vi "Phasor Compute f(tau) & Zeros.vi"(0 "f(tau) Graph Refnum":refnum<vi>, 1 "Phasor Graph Refnum":refnum<vi>, 5 "Phasor Parameters":T1={"Display Parameters"={"# Points"=0, "Ramp Type"=enum."Linear", "Type of Series"=enum."1-Exp Decays", "Min tau"=0.0, "Max tau"=0.0, "Include 0"=FALSE, "Include Infinity"=FALSE}, "Phasor Parameters"={"Harmonic Frequency"=0.0, "Use f* = 1/D Frequency"=FALSE, "Calibrated Phasor"=FALSE, "Calibration Lifetime"=1e-09, "Phasor Calculation"=enum."Direct Sum", "SEPL Type"=enum."UC", "# Gates"=1.0, "Square Gate Width"=1e-09, "Show Ticks"=FALSE}, "Decay & IRF Parameters"={"Lifetime"=0.0, "IRF Offset"=0.0, "IRF Period"=0.0, "Normalized Decays"=FALSE, "IRF Model"=enum."Dirac", "IRF Parameter 1"=0.0}, "Gate Parameters"={"First Gate Start"=0.0, "Use Gate Center"=FALSE, "Gate Width"=0.0, "Gate Step"=0.0, "# Gates"=0.0, "Gate Type"=enum."Square", "Edge Width"=0.0, "Top Slope"=0.0, "Reversed Sawtooth?"=FALSE, "Analytical Computation"=FALSE, "Integration"=enum."Item 0", "Tolerance"=1.0, "# Steps"=1.0, "Type of User-defined Function"=enum."Gate", "Use Gate Step"=FALSE}, "Detector Parameters"={"Frames/Image"=0, "Gates/Frame"=0, "Bits/Frame"=0, "Multiplicity"=0, "Incident Signal"=0.0, "Poisson Signal"=FALSE}} {"Detector Parameters"."Frames/Image" min=1; "Detector Parameters"."Multiplicity" min=0; "Detector Parameters"."Bits/Frame" min=1; "Detector Parameters"."Gates/Frame" min=1; "Gate Parameters"."# Steps" min=0.0; "Gate Parameters"."Tolerance" min=0.0; "Gate Parameters"."Top Slope" min=0.0; "Gate Parameters"."Edge Width" min=0.0; "Gate Parameters"."Gate Step" min=0.0; "Gate Parameters"."# Gates" min=0.0 step=1.0; "Gate Parameters"."Gate Width" min=0.0; "Decay & IRF Parameters"."Lifetime" min=0.0; "Decay & IRF Parameters"."IRF Period" min=0.0; "Phasor Parameters"."Square Gate Width" min=0.0; "Phasor Parameters"."# Gates" min=0.0; "Phasor Parameters"."Calibration Lifetime" min=0.0; "Phasor Parameters"."Harmonic Frequency" min=0.0; "Display Parameters"."Min tau" min=0.0; "Display Parameters"."Max tau" min=0.0; "Display Parameters"."# Points" min=1 step=1}, 7 "Linear Coefficients":cluster{"u":dbl, "v":dbl}, 11 "Error In":errorcluster, 12 "Use Cursor":bool) -> (4 "Numerical Solution 1":dbl[unit], 6 "Numerical Solution 2":dbl[unit], 8 "Analytical Solution 1":dbl[unit], 10 "Analytical Solution 2":dbl[unit], 15 "Error Out":errorcluster)   [LabVIEW 2021, in "Phasor.lvlib"]
uses:
  Phasor.lvlib
  Phasor SEPL Parameters.ctl
  Phasor Explorer Display Parameters.ctl
  Phasor Type of Series.ctl
  Phasor Explorer Phasor Parameters.ctl
  Phasor Calculation Type.ctl
  Phasor SEPL Type.ctl
  Phasor Explorer Decay Parameters.ctl
  Phasor IRF Model.ctl
  Phasor Explorer Gate Parameters.ctl
  Phasor Gate Type.ctl
  Phasor Type of User-defined Function.ctl
  Phasor Explorer Detector Parameters.ctl
  Phasor Explorer f(tau) [SEPL Intersections].vi
  <vilib>/gmath/zero.llb/Find All Zeros of f(x) (VI).vi
  <vilib>/ErrorRing/Error Ring.xnode
  Image/Image.lvlib
  <vilib>/gmath/NI_Gmath.lvlib
  Phasor Explorer.lvlib
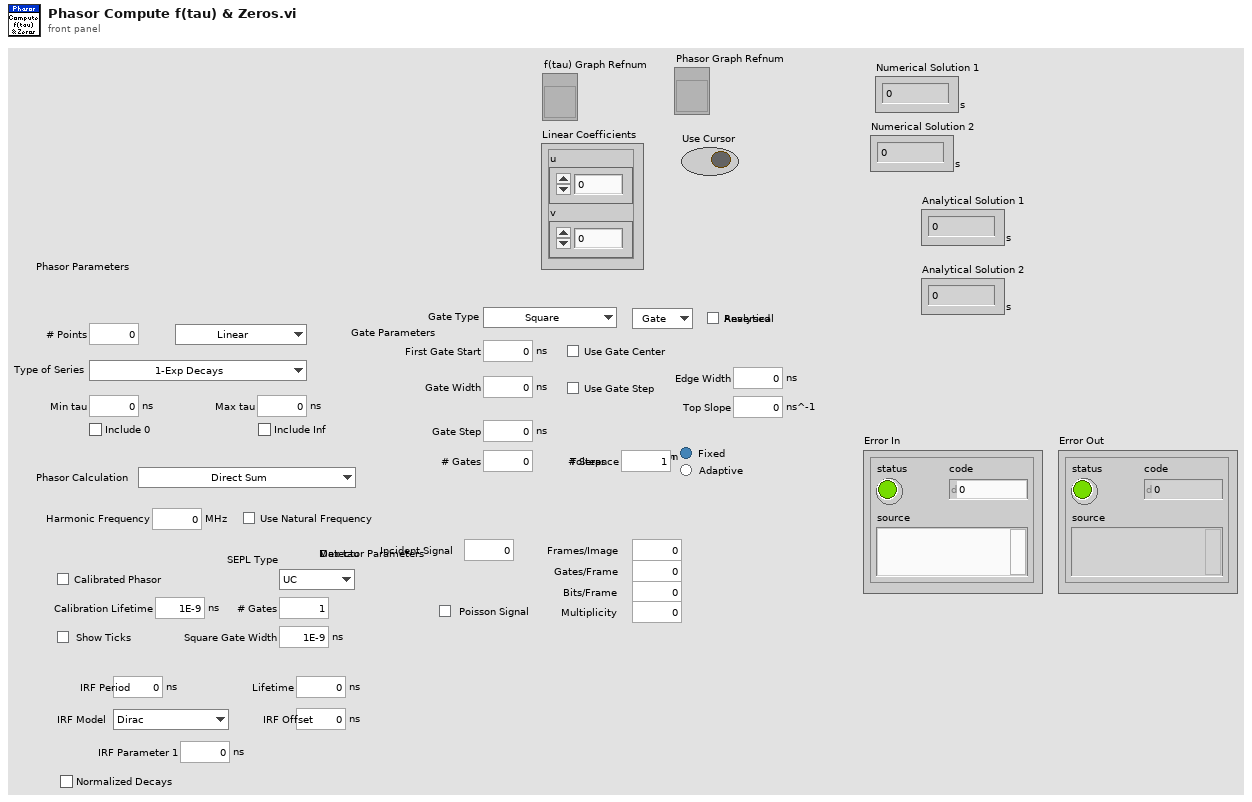
[diagram p1: front panel]
types:
  T1 = typedef "Phasor.lvlib/Phasor SEPL Parameters.ctl" = cluster{"Display Parameters":T2, "Phasor Parameters":T4, "Decay & IRF Parameters":T7, "Gate Parameters":T9, "Detector Parameters":T12}
  T2 = typedef "Phasor Explorer.lvlib/Phasor Explorer Display Parameters.ctl" = cluster{"# Points":i32, "Ramp Type":enum16{"Linear", "Logarithmic"}, "Type of Series":T3, "Min tau":dbl[unit], "Max tau":dbl[unit], "Include 0":bool, "Include Infinity":bool}
  T3 = typedef "Phasor.lvlib/Phasor Type of Series.ctl" = enum16{"1-Exp Decays", "Linear Combination of 1-Exp"}
  T4 = typedef "Phasor Explorer.lvlib/Phasor Explorer Phasor Parameters.ctl" = cluster{"Harmonic Frequency":dbl[unit], "Use f* = 1/D Frequency":bool, "Calibrated Phasor":bool, "Calibration Lifetime":dbl[unit], "Phasor Calculation":T5, "SEPL Type":T6, "# Gates":dbl, "Square Gate Width":dbl[unit], "Show Ticks":bool}
  T5 = typedef "Phasor.lvlib/Phasor Calculation Type.ctl" = enum16{"Direct Sum", "Analytical Formula"}
  T6 = typedef "Phasor.lvlib/Phasor SEPL Type.ctl" = enum16{"UC", "L_N", "L_N[W]", "L_X"}
  T7 = typedef "Phasor Explorer.lvlib/Phasor Explorer Decay Parameters.ctl" = cluster{"Lifetime":dbl[unit], "IRF Offset":dbl[unit], "IRF Period":dbl[unit], "Normalized Decays":bool, "IRF Model":T8, "IRF Parameter 1":dbl[unit]}
  T8 = typedef "Phasor.lvlib/Phasor IRF Model.ctl" = enum16{"Dirac", "Exponential"}
  T9 = typedef "Phasor Explorer.lvlib/Phasor Explorer Gate Parameters.ctl" = cluster{"First Gate Start":dbl[unit], "Use Gate Center":bool, "Gate Width":dbl[unit], "Gate Step":dbl[unit], "# Gates":dbl, "Gate Type":T10, "Edge Width":dbl[unit], "Top Slope":dbl[unit], "Reversed Sawtooth?":bool, "Analytical Computation":bool, "Integration":enum32{"Item 0", "Item 1"}, "Tolerance":dbl, "# Steps":dbl, "Type of User-defined Function":T11, "Use Gate Step":bool}
  T10 = typedef "Phasor.lvlib/Phasor Gate Type.ctl" = enum16{"Square", "Finite Edge Square", "Finite Edge, Tilted Top Square", "Triangle", "Sawtooth", "User-defined"}
  T11 = typedef "Phasor.lvlib/Phasor Type of User-defined Function.ctl" = enum16{"Gate", "IRF"}
  T12 = typedef "Phasor Explorer.lvlib/Phasor Explorer Detector Parameters.ctl" = cluster{"Frames/Image":i32, "Gates/Frame":i32, "Bits/Frame":i32, "Multiplicity":i32, "Incident Signal":dbl, "Poisson Signal":bool}
  T13 = typedef "LVCursorListTypeDef.ctl" = cluster{"Name":string, "Color":u32, "Style":u8, "Point Style":u8, "Name Visible":bool, "Allow Drag":bool, "Cursor Mode":u32, "Plot":i32, "Index":i32, "Position":cluster{"X":dbl, "Y":dbl}, "X Scale":u32, "Y Scale":u32, "Watch Plots":i32[], "Watch All Plots":bool, "Plot Area":i32, "Label Offset":cluster{"X":dbl, "Y":dbl}}[]
  T14 = cluster{"Name":string, "Color":u32, "Style":u8, "Point Style":u8, "Name Visible":bool, "Allow Drag":bool, "Cursor Mode":u32, "Plot":i32, "Index":i32, "Position":cluster{"X":dbl, "Y":dbl}, "X Scale":u32, "Y Scale":u32, "Watch Plots":i32[], "Watch All Plots":bool, "Plot Area":i32, "Label Offset":cluster{"X":dbl, "Y":dbl}}
  T15 = typedef "Phasor.lvlib/Phasor Data for SEPL Intersections.ctl" = cluster{"Linear Coefficients":cluster{"u":dbl, "v":dbl}, "Decay Definition":T16, "Gates Definitions":T17, "iw":cdb, "Phasor Calculation":T5}
  T16 = typedef "Phasor.lvlib/Phasor Decay Definiton.ctl" = cluster{"offset: t0":ext, "period: T":ext, "lifetime: tau":ext, "Incident Signal: I":ext, "Normalized Decays":bool, "IRF Model":T8, "IRF Parameter 1":ext, "Poisson Signal":bool}
  T17 = typedef "Phasor.lvlib/Phasor Gate Definitions.ctl" = cluster{"First Gate: t1":ext, "Gate Width: W":ext, "Gate Step: d":ext, "# Gates: G":ext, "Use Gate Center":bool, "Frames/Image: F":i32, "Gates/Frame: L":i32, "Bits/Frame: q":i32, "Multiplicity: p":i32, "Gate Type":T10, "Gate Edge s":ext, "Gate Top Slope":ext, "Reversed Sawtooth?":bool, "Computation":bool, "User-defined Gate":T18, "Tolerance":ext, "Integration":enum32{"Item 0", "Item 1"}, "# Steps":ext, "Type of User-defined Function":enum32{"Gate", "IRF"}}
  T18 = typedef "XY Graph Add-Ons.lvlib/XY Plot Data.ctl" = cluster{"X Array":dbl[], "Y Array":dbl[]}
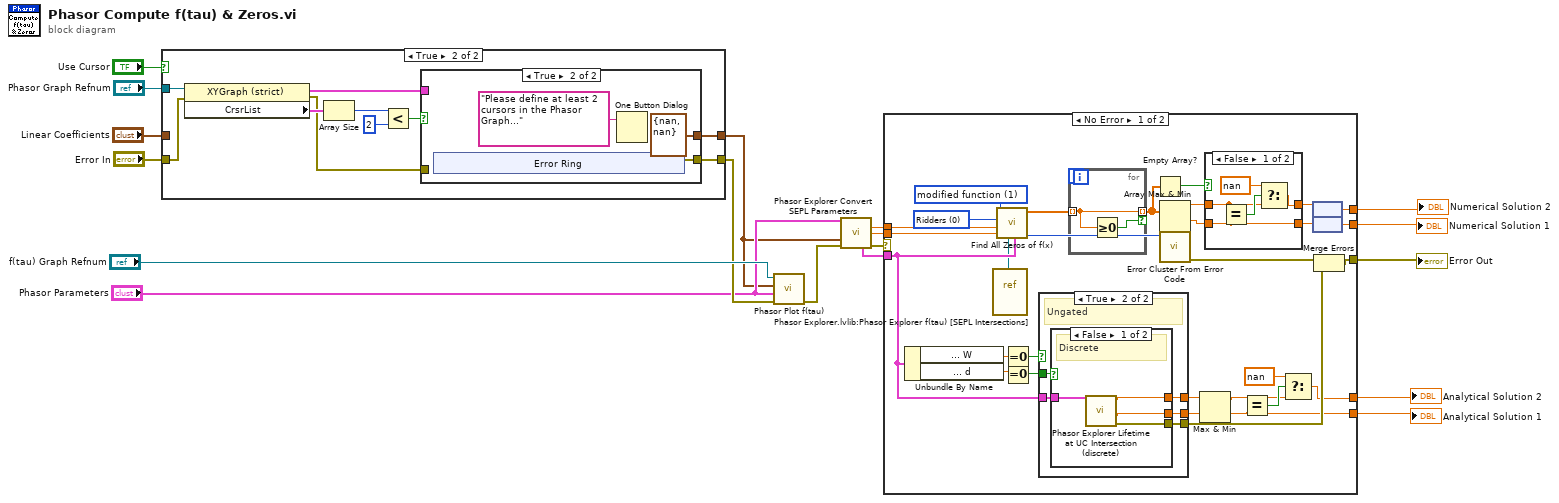
[diagram p0: block diagram]
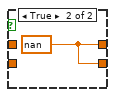
[diagram p2: hidden frame]
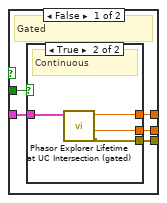
[diagram p3: hidden frame]
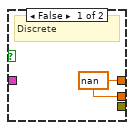
[diagram p4: hidden frame]
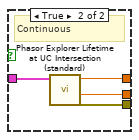
[diagram p5: hidden frame]
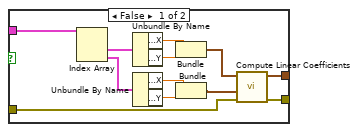
[diagram p8: hidden frame]
diagram:
  n1 = case shown="True" "Use Cursor" {
    tunnel: "Phasor Graph Refnum" -> [_ w29]
    tunnel: [w20 w24] -> w5
    tunnel: "Linear Coefficients" -> [w20 _]
    tunnel: "Error In" -> [w19 w23]
    tunnel: [w19 w21] -> w13
    frame False {
    }
    frame True {
      n2 = property class="XYGraph (strict)"(reference=w29, error in=w23) -> (error out=w22:errorcluster, "CrsrList"=w25:T13)  [unwired: 1 out]
      n3 = Array Size(array=w25) -> (size(s)=w28:i32)
      n4 = Less?(x=w28, y=2) -> (x < y?=w26:bool)
      n5 = case shown="True" w26 {
        tunnel: w25 -> [w41 _]
        tunnel: [w33 cluster{"u":dbl, "v":dbl} {"u"=nan, "v"=nan} ("Linear Coefficients")] -> w24
        tunnel: w22 -> [w31 _]
        tunnel: [w30 w42] -> w21
        frame False {
          n6 = Index Array(array=w41) -> (element #1=w40:T14, element #2=w39:T14)  [unwired: 2 in]
          n7 = Unbundle By Name(w40) -> ("Position.X"=w38:dbl, "Position.Y"=w37:dbl)
          n8 = Unbundle By Name(w39) -> ("Position.X"=w35:dbl, "Position.Y"=w34:dbl)
          n9 = Bundle("X"=w38, "Y"=w37) -> (w36:cluster{"X":dbl, "Y":dbl})  [unwired: 1 in]
          n10 = Bundle("X"=w35, "Y"=w34) -> (w32:cluster{"X":dbl, "Y":dbl})  [unwired: 1 in]
          n11 = call "Compute Linear Coefficients.vi"("Error In"=w31, "Point 2"=w32, "Point 1"=w36) -> ("Error Out"=w30:errorcluster, "Linear Coefficients"=w33:cluster{"u":dbl, "v":dbl})  [unwired: 7 in]
        }
        frame True {
          n12 = xnode "Error Ring"() -> ("error out"=w42:errorcluster)
          n13 = One Button Dialog(message="Please define at least 2 cursors in the Phasor Graph...") -> ()  [unwired: 1 in, 1 out]
        }
      }
    }
  }
  n14 = call "Phasor Plot f(tau).vi"("error in (no error)"=w13, "Phasor Parameters"="Phasor Parameters", "Linear Coefficients"=w5, "XYGraph in"="f(tau) Graph Refnum") -> ("error out"=w11:errorcluster)  [unwired: 7 in]
  n15 = call "Phasor Explorer Convert SEPL Parameters.vi"("Phasor Parameters"="Phasor Parameters", "Linear Coefficients"=w5, "Error In"=w11) -> ("Min tau"=w9:dbl, "Max tau"=w8:dbl, "Data for Pseudo UC Intersections"=w7:T15, "Error Out"=w10:errorcluster)  [unwired: 7 in, 2 out]
  n16 = case shown="No Error" w10 {
    selector: w10 -> [_ w110]
    tunnel: w9 -> [w76 _]
    tunnel: w8 -> [w75 _]
    tunnel: w7 -> [w66 _]
    tunnel: [w65 w110] -> w6
    tunnel: [w72 _] -> w4
    tunnel: [w71 _] -> w3
    tunnel: [w53 _] -> w2
    tunnel: [w49 _] -> w1
    frame No Error {
      w77 = u16 1 items=["fixed function", "modified function"] ("step type")
      w78 = u16 0 items=["Ridders", "Newton Raphson"] ("algorithm")
      n17 = Unbundle By Name(w66) -> ("Gates Definitions.Gate Width: W"=w70:ext, "Gates Definitions.Gate Step: d"=w69:ext)
      n18 = vi-ref "Phasor Explorer.lvlib:Phasor Explorer f(tau) [SEPL Intersections].vi"() -> (w63:refnum<vi>)
      n19 = call-poly <vilib>:"Find All Zeros of f(x).vi"("data"=w66, "f(x)"=w63, "end"=w75, "start"=w76, "algorithm"=w78, "step type"=w77) -> ("error"=w74:i32, "Zeros"=w62:dbl[])  [unwired: 2 in, 2 out]
      n20 = Equal To 0?(x=w70) -> (x = 0?=w68:bool)
      n21 = Equal To 0?(x=w69) -> (x = 0?=w67:bool)
      n22 = case shown="True" w68 {
        tunnel: w67 -> [w91 w101]
        tunnel: w66 -> [w90 w100]
        tunnel: [w88 w99] -> w52
        tunnel: [w87 w98] -> w51
        tunnel: [w89 w97] -> w64
        frame False {
          # "Gated"
          n23 = case shown="True" w91 {
            tunnel: w90 -> [_ w96]
            tunnel: [_ w95] -> w89
            tunnel: [w92 w94] -> w88
            tunnel: [w92 w93] -> w87
            frame False {
              w92 = dbl[unit] nan ("Analytical Solution 2")
              # "Discrete"
            }
            frame True {
              # "Continuous"
              n24 = call "Phasor Explorer Lifetime at UC Intersection (gated).vi"("Data for Pseudo UC Intersections"=w96) -> ("Error Out"=w95:errorcluster, "Analytical Solution 1"=w93:dbl[unit], "Analytical Solution 2"=w94:dbl[unit])  [unwired: 8 in]
            }
          }
        }
        frame True {
          # "Ungated"
          n25 = case shown="False" w101 {
            tunnel: w100 -> [w105 w109]
            tunnel: [w104 w108] -> w99
            tunnel: [w103 w107] -> w98
            tunnel: [w102 w106] -> w97
            frame False {
              # "Discrete"
              n26 = call "Phasor Explorer Lifetime at UC Intersection (discrete).vi"("Data for Pseudo UC Intersections"=w105) -> ("Error Out"=w102:errorcluster, "Analytical Solution 1"=w103:dbl[unit], "Analytical Solution 2"=w104:dbl[unit])  [unwired: 8 in]
            }
            frame True {
              # "Continuous"
              n27 = call "Phasor Explorer Lifetime at UC Intersection (standard).vi"("Data for Pseudo UC Intersections"=w109) -> ("Error Out"=w106:errorcluster, "Analytical Solution 1"=w107:dbl[unit], "Analytical Solution 2"=w108:dbl[unit])  [unwired: 8 in]
            }
          }
        }
      }
      n28 = for {
        tunnel: w62 -> [w86] mode=indexing
        tunnel: [w86] -> w61 mode=indexing if=w85
        n29 = Greater Or Equal To 0?(x=w86) -> (x >= 0?=w85:bool)
      }
      n30 = Empty Array?(array=w61) -> (empty?=w60:bool)
      n31 = Array Max & Min(array=w61) -> (max value=w59:dbl, min value=w58:dbl)  [unwired: 2 out]
      n32 = call <vilib>:"Error Cluster From Error Code.vi"("error code (0)"=w74) -> ("error out"=w73:errorcluster)  [unwired: 8 in]
      n33 = Max & Min(x=w52, y=w51) -> (max(x,y)=w50:dbl[unit], min(x,y)=w49:dbl[unit])
      n34 = case shown="False" w60 {
        tunnel: w59 -> [w81 _]
        tunnel: w58 -> [w83 _]
        tunnel: [w83 w84] -> w57
        tunnel: [w79 w84] -> w56
        frame False {
          n35 = Equal?(x=w81, y=w83) -> (x = y?=w82:bool)
          n36 = Select(t=nan, s=w82, f=w81) -> (s? t:f=w79:dbl)
        }
        frame True {
          w84 = nan
        }
      }
      n37 = Equal?(x=w50, y=w49) -> (x = y?=w54:bool)
      n38 = Select(t=nan, s=w54, f=w50) -> (s? t:f=w53:dbl[unit])
      n39 = node(w56) -> (w72:dbl[unit])
      n40 = node(w57) -> (w71:dbl[unit])
      n41 = Merge Errors(w73, w64) -> (w65:errorcluster)
    }
    frame Error {
    }
  }
  "Numerical Solution 2" <- w4
  "Numerical Solution 1" <- w3
  "Error Out" <- w6
  "Analytical Solution 2" <- w2
  "Analytical Solution 1" <- w1
